vi "禹山过程全局变量.vi"() -> ()   [LabVIEW 2016, in "斯坦道多参数.lvlib"]
panel:
  out "DO 2":cluster{"温度测量值":sgl, "DO%":sgl, "DOmg/L":sgl}
  out "spcond":cluster{"温度测量值":sgl, "测量值":sgl, "错误标志":u16} {"错误标志" items=["NO Error"=0, "量程切换错误标识"=255]}
  out "pH":cluster{"温度测量值":sgl, "ORP":sgl, "pH":sgl}
  out "浊度":cluster{"温度测量值":sgl, "浊度测量值":sgl}
  out "DO":cluster{"温度测量值":sgl, "DO%":sgl, "DOmg/L":sgl}
  out "叶绿素a":cluster{"温度测量值":sgl, "叶绿素测量值":sgl, "错误标志":u16} {"错误标志" items=["NO Error"=0, "刷子没到位"=255]}
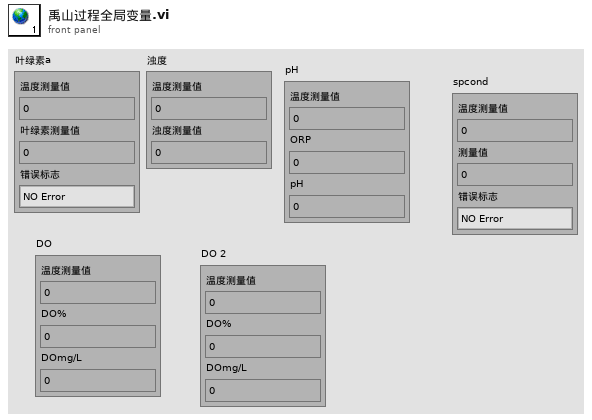
[diagram p1: front panel]
diagram:
